vi "PIDINIT.vi"(11 "setpoint":dbl format="%.2f") -> ()   [LabVIEW 2013]
uses:
  <vilib>/addons/control/pid/pid.llb/PID (DBL).vi
  <vilib>/addons/control/pid/NI_PID_pid.lvlib
panel:
  in  "y 2":dbl=0.59
  in  "PID Gains for distance":T1={"proportional gain (Kc)"=1.0, "integral time (Ti, min)"=0.01, "derivative time (Td, min)"=0.0} {"derivative time (Td, min)" format="%.3f"; "integral time (Ti, min)" format="%.3f"; "proportional gain (Kc)" format="%.3f"}
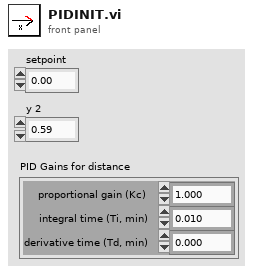
[diagram p1: front panel]
types:
  T1 = cluster{"proportional gain (Kc)":dbl, "integral time (Ti, min)":dbl, "derivative time (Td, min)":dbl}
  T2 = typedef "WPI_EncoderDevRef.ctl" = cluster{"DevStatus":errorcluster, "EncoderIndex":T3, "CounterIndex":T4, "DistancePerCount":dbl, "Decoding Type":T5}
  T3 = typedef "FPGA_EncoderIdx.ctl" = enum8{"Enc 0", "Enc 1", "Enc 2", "Enc 3", "Invalid"}
  T4 = typedef "FPGA_CounterCtrSystemIndex.ctl" = enum8{"Ctr 0", "Ctr 1", "Ctr 2", "Ctr 3", "Ctr 4", "Ctr 5", "Ctr 6", "Ctr 7", "Invalid"}
  T5 = typedef "WPI_EncoderType.ctl" = enum16{"1x", "2x", "4x"}
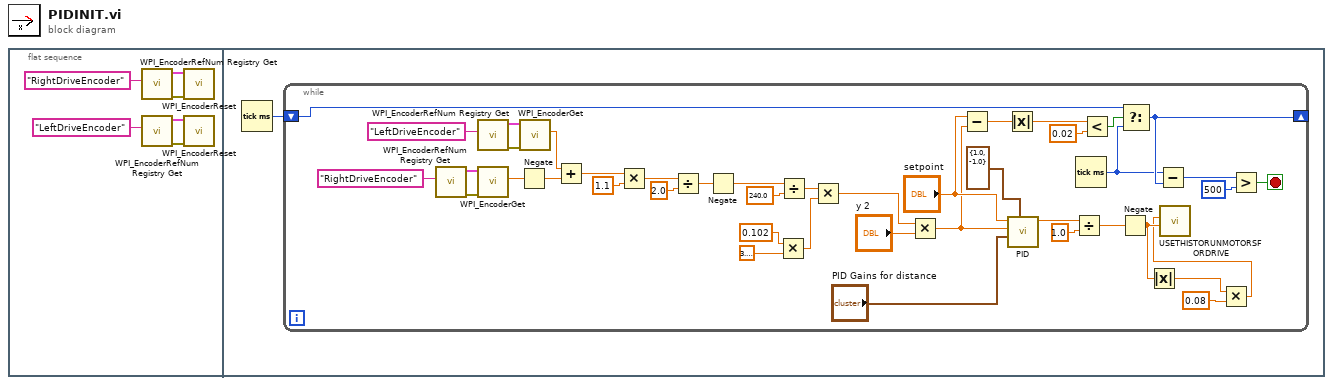
[diagram p0: block diagram]
diagram:
  n1 = flat-sequence {
    frame #0 {
      n2 = call <vilib>:"WPI_EncoderRefNum Registry Get.vi"("refnum name"="RightDriveEncoder") -> ("error out"=w5:errorcluster, "EncoderDevRef"=w6:T2)  [unwired: 9 in]
      n3 = call <vilib>:"WPI_EncoderRefNum Registry Get.vi"("refnum name"="LeftDriveEncoder") -> ("error out"=w3:errorcluster, "EncoderDevRef"=w4:T2)  [unwired: 9 in]
      n4 = call <vilib>:"WPI_EncoderReset.vi"("error in (no error)"=w5, "EncoderDevRef"=w6) -> ()  [unwired: 8 in, 2 out]
      n5 = call <vilib>:"WPI_EncoderReset.vi"("error in (no error)"=w3, "EncoderDevRef"=w4) -> ()  [unwired: 8 in, 2 out]
    }
    frame #1 {
      n6 = Tick Count (ms)() -> (millisecond timer value=w7:u32)
      n7 = while {
        shift-right: [w24] -> _
        shift-left: w7 -> [w25]
        stop <- w20 stop-if-true
        n8 = call <vilib>:"WPI_EncoderRefNum Registry Get.vi"("refnum name"="RightDriveEncoder") -> ("error out"=w48:errorcluster, "EncoderDevRef"=w47:T2)  [unwired: 9 in]
        n9 = call <vilib>:"WPI_EncoderRefNum Registry Get.vi"("refnum name"="LeftDriveEncoder") -> ("error out"=w50:errorcluster, "EncoderDevRef"=w49:T2)  [unwired: 9 in]
        n10 = call <vilib>:"WPI_EncoderGet.vi"("error in (no error)"=w48, "EncoderDevRef"=w47) -> ("Distance"=w18:dbl)  [unwired: 4 in, 5 out]
        n11 = Negate(x=w18) -> (-x=w17:dbl)
        n12 = call <vilib>:"WPI_EncoderGet.vi"("error in (no error)"=w50, "EncoderDevRef"=w49) -> ("Distance"=w44:dbl)  [unwired: 4 in, 5 out]
        n13 = Add(x=w44, y=w17) -> (x+y=w14:dbl)
        n14 = Multiply(x=w14, y=1.1) -> (x*y=w12:dbl)
        n15 = Divide(x=w12, y=2.0) -> (x/y=w16:dbl)
        n16 = Negate(x=w16) -> (-x=w15:dbl)
        n17 = Multiply(x=0.102, y=3.141592653589793) -> (x*y=w39:dbl)
        n18 = Divide(x=w15, y=240.0) -> (x/y=w37:dbl)
        n19 = Multiply(x=w37, y=w39) -> (x*y=w34:dbl)
        n20 = Multiply(x=w34, y="y 2") -> (x*y=w30:dbl)
        n21 = Subtract(x="setpoint", y=w30) -> (x-y=w29:dbl)
        n22 = Absolute Value(x=w29) -> (abs(x)=w28:dbl)
        n23 = call-poly <vilib>:"PID.vi"("output range"=cluster{"output high":dbl, "output low":dbl} {"output high"=1.0, "output low"=-1.0}, "PID gains"="PID Gains for distance", "process variable"=w30, "setpoint"="setpoint") -> ("output"=w38:dbl)  [unwired: 6 in, 1 out]
        n24 = Divide(x=w38, y=1.0) -> (x/y=w19:dbl)
        n25 = Tick Count (ms)() -> (millisecond timer value=w23:u32)
        n26 = Less?(x=w28, y=0.02) -> (x < y?=w26:bool)
        n27 = Negate(x=w19) -> (-x=w11:dbl)
        n28 = Select(t=w25, s=w26, f=w23) -> (s? t:f=w24:u32)
        n29 = Absolute Value(x=w11) -> (abs(x)=w9:dbl)
        n30 = Subtract(x=w23, y=w24) -> (x-y=w22:u32)
        n31 = Multiply(x=w9, y=0.08) -> (x*y=w8:dbl)
        n32 = call "USETHISTORUNMOTORSFORDRIVE.vi"("Y axis value"=w11, "X axis value"=w8) -> ()  [unwired: 10 in]
        n33 = Greater?(x=w22, y=u32 500) -> (0:w20:bool)
      }
    }
  }
